vi "Omni Robot Model.vi"(10 "reset":bool, 11 "motor ccw velocity setpoint":dbl[](array[numeric])=[0.0, 0.0, 0.0]) -> (2 "robot position":T1, 3 "motor ccw angular velocities":dbl[](array[numeric]))   [LabVIEW 2015]
uses:
  Robot Position.ctl
  Motor Velocity PID.vi
  Motor Model.vi
  Omni Robot Body Model.vi
  <vilib>/Simulation/Implementation/Shared/SIMSCR Execution Mode.ctl
  <vilib>/Simulation/Scripting/Companion Diagram/SimConfigNode/SimParams.ctl
  <vilib>/Simulation/Scripting/Companion Diagram/SimConfigNode/_simSolvers.ctl
  <vilib>/Simulation/Param Hierarchy/Typedefs/SIMPH Param Control Actions.ctl
  <vilib>/Simulation/Implementation/Shared/NILVSim_ParamChanged.vi
  <vilib>/Simulation/Implementation/Shared/NILVSIM_BeginStep.vi
  <vilib>/Simulation/SignalArithmetic/Implementation/NILVSim Gain.llb/SIM Gain (vector).vi
  <vilib>/Simulation/Implementation/Shared/NILVSim_Manager.vi
  <vilib>/Utility/error.llb/Clear Errors.vi
  <vilib>/Simulation/Implementation/Shared/NILVSim_FinalizeModel.vi
  <vilib>/Simulation/Implementation/Shared/SIM Unbundle Sim Info.vi
  <vilib>/Simulation/Implementation/Shared/SIMSH Read Queue.vi
  <vilib>/Simulation/Implementation/Shared/NILVSim_Initialize.vi
  <vilib>/Simulation/Utility/Implementation/NILVSim Get Time and IsAcceptedStep.vi
  <vilib>/Simulation/Implementation/Shared/NILVSim_GetModelError.vi
  <vilib>/Simulation/Implementation/Shared/SIM SimErrorHandler.vi
  <vilib>/Simulation/Implementation/Shared/SIM Bundle Sim Info.vi
  <vilib>/Simulation/Scripting/Companion Diagram/SimConfigNode/SimDog.xnode
  <vilib>/Simulation/Implementation/XNodeFramework/SimXNode/SimX.xnode
  <vilib>/Simulation/Implementation/Shared/NI_SIM_Implementation.lvlib
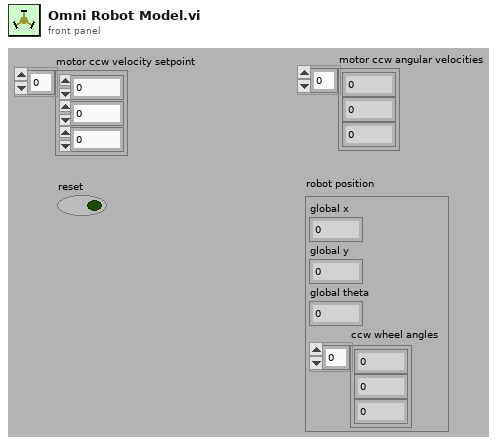
[diagram p1: front panel]
types:
  T1 = typedef "Robot Position.ctl" = cluster{"global x":dbl, "global y":dbl, "global theta":dbl, "ccw wheel angles":dbl[]}
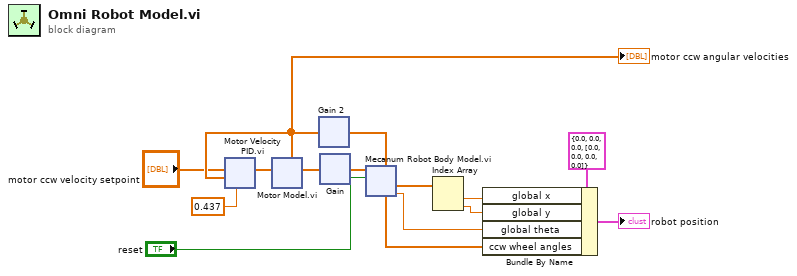
[diagram p0: block diagram]
diagram:
  n1 = xnode ("Motor Velocity PID.vi")("DC current max"=0.437, "ccw velocity process variable"=w11, "ccw velocity setpoint"="motor ccw velocity setpoint") -> ("DC current output"=w12:dbl[])  [unwired: 3 in, 5 out]
  n2 = xnode ("Motor Model.vi")("motor angular velocity"=w11, "DC current"=w12) -> ("motor torque"=w15:dbl[])  [unwired: 1 in, 8 out]
  n3 = xnode ("Gain")("input"=w15) -> ("output"=w14:dbl[])  [unwired: 3 in]
  n4 = xnode ("Mecanum Robot Body Model.vi")("reset"="reset", "ccw torques"=w14) -> ("theta 2"=w5:dbl, "x,y (inertial)"=w6:dbl[], "ccw wheel angles"=w4:dbl[], "ccw wheel angular velocities"=w13:dbl[])  [unwired: 6 out]
  n5 = xnode ("Gain 2")("input"=w13) -> ("output"=w11:dbl[])  [unwired: 3 in]
  "motor ccw angular velocities" <- w11
  n6 = Index Array(array=w6) -> (element #1=w8:dbl, element #2=w7:dbl)  [unwired: 2 in]
  n7 = Bundle By Name(cluster=T1 {"global x"=0.0, "global y"=0.0, "global theta"=0.0, "ccw wheel angles"=[0.0, 0.0, 0.0, 0.0]} ("robot position 2"), "global x"=w8, "global y"=w7, "global theta"=w5, "ccw wheel angles"=w4) -> (→"robot position":T1)
